vi "Supervisório Comunicação RS485.vi"() -> ()   [LabVIEW 2013]
uses:
  <vilib>/Instr/_visa.llb/VISA Configure Serial Port (Instr).vi
panel:
  in  "?":enum32{"Dados", "Gráficos"}(tab)
  out "MENSAGENS DO CONTROLADOR":string
  out "MENSAGENS DO INVERSOR":string
  out "POTENCIA SAIDA":dbl
  out "TEMPERATURA":dbl
  in  "?":bool
  in  "?":dbl(knob) scale=0.0..99.0
  in  "?":bool
  in  "?":bool
  out "STATUS DO INVERSOR":dbl
  out "POTÊNCIA DE SAÍDA [W]":dbl
  out "DC LINK [Vdc]":dbl
  out "TENSÃO DE SAÍDA [Vac]":dbl
  out "FREQUENCIA SAIDA [Hz]":dbl
  out "CORRENTE SAÍDA [A]":dbl
  in  "?":bool
  in  "Baud Rate":u32=9600
  in  "PORTA COM":refnum<visa-resource-name>
  out "?":i32(graph)
  out "?":i32(graph)
  out "?":dbl(graph)
  out "?":dbl(graph)
  out "?":dbl
  out "?":dbl
  out "?":dbl
  out "?":dbl
  # "Configura Serial"
  # "Dados do inversor"
  # "Dados temperatura"
  # "Frequencia de operação inversor"
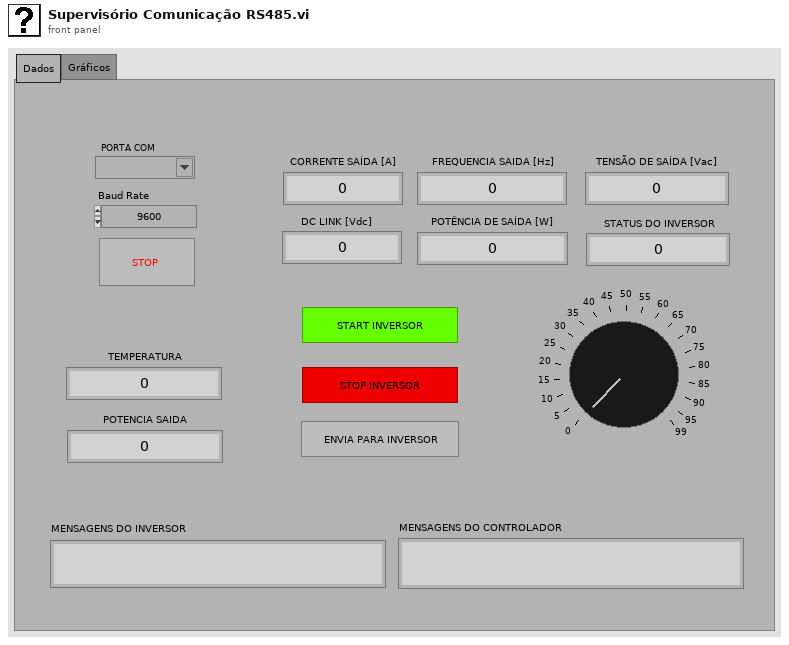
[diagram p1: front panel]
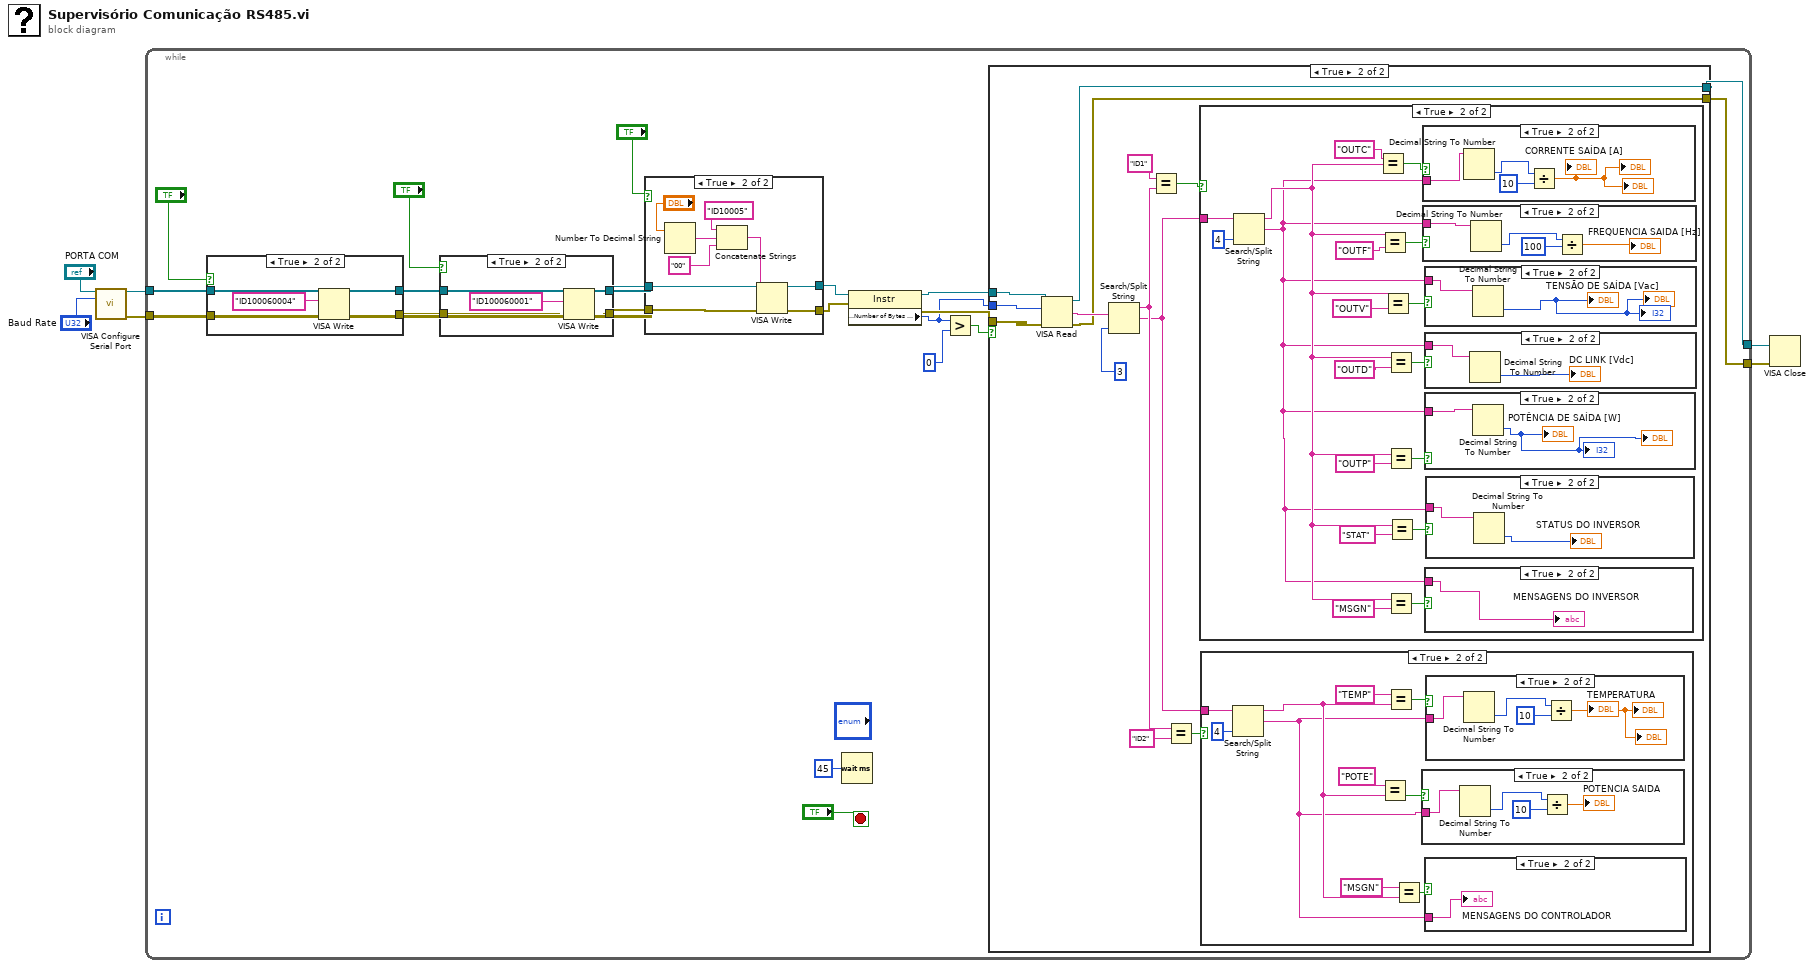
[diagram p0: block diagram]
diagram:
  n1 = call-poly "VISA Configure Serial Port"("VISA resource name"="PORTA COM", "baud rate (9600)"="Baud Rate") -> ("VISA resource name out"=w5:refnum<visa-resource-name>, "error out"=w4:errorcluster)  [unwired: 12 in]
  n2 = while {
    tunnel: w5 -> [w10]
    tunnel: w4 -> [w9]
    tunnel: [w20] -> w2
    tunnel: [w19] -> w1
    stop <- "?" stop-if-true
    n3 = case shown="True" "?" {
      tunnel: w10 -> [w28 w31]
      tunnel: w9 -> [w27 w30]
      tunnel: [w28 w32] -> w11
      tunnel: [w27 w29] -> w12
      frame False {
      }
      frame True {
        n4 = VISA Write(VISA resource name=w31, write buffer="ID100060004", error in (no error)=w30) -> (VISA resource name out=w32:refnum<visa-resource-name>, error out=w29:errorcluster)  [unwired: 1 out]
      }
    }
    n5 = case shown="True" "?" {
      tunnel: w11 -> [w46 w51]
      tunnel: w12 -> [w45 w50]
      tunnel: [w46 w48] -> w16
      tunnel: [w45 w47] -> w15
      frame False {
      }
      frame True {
        n6 = VISA Write(VISA resource name=w51, write buffer="ID100060001", error in (no error)=w50) -> (VISA resource name out=w48:refnum<visa-resource-name>, error out=w47:errorcluster)  [unwired: 1 out]
      }
    }
    n7 = case shown="True" "?" {
      tunnel: w16 -> [w35 w43]
      tunnel: w15 -> [w34 w42]
      tunnel: [w35 w37] -> w14
      tunnel: [w34 w36] -> w13
      frame False {
      }
      frame True {
        n8 = Number To Decimal String(number="?") -> (decimal integer string=w39:string)  [unwired: 1 in]
        n9 = Concatenate Strings("ID10005" ("string"), w39, "00" ("string")) -> (w41:string)
        n10 = VISA Write(VISA resource name=w43, write buffer=w41, error in (no error)=w42) -> (VISA resource name out=w37:refnum<visa-resource-name>, error out=w36:errorcluster)  [unwired: 1 out]
      }
    }
    n11 = Wait (ms)(milliseconds to wait=u32 45) -> ()  [unwired: 1 out]
    n12 = property class="Instr"(reference=w14, error in=w13) -> (reference out=w24:refnum<visa-resource-name>, error out=w23:errorcluster, "Serial Settings:Number of Bytes at Serial Port"=w22:u32)
    n13 = Greater?(x=w22, y=u32 0) -> (0:w25:bool)
    n14 = case shown="True" w25 {
      tunnel: w24 -> [w53 w55]
      tunnel: w23 -> [w52 w57]
      tunnel: w22 -> [_ w66]
      tunnel: [w53 w54] -> w20
      tunnel: [w52 w56] -> w19
      frame False {
      }
      frame True {
        n15 = VISA Read(VISA resource name=w55, byte count=w66, error in (no error)=w57) -> (VISA resource name out=w54:refnum<visa-resource-name>, read buffer=w65:string, error out=w56:errorcluster)  [unwired: 1 out]
        n16 = Search/Split String(string=w65, offset (0)=3) -> (substring before match=w60:string, match + rest of string=w58:string)  [unwired: 1 in, 1 out]
        n17 = Equal?(x="ID1", y=w60) -> (x = y?=w62:bool)
        n18 = Equal?(x=w60, y="ID2") -> (x = y?=w61:bool)
        n19 = case shown="True" w62 {
          tunnel: w58 -> [_ w103]
          frame False {
          }
          frame True {
            n20 = Search/Split String(string=w103, offset (0)=4) -> (substring before match=w87:string, match + rest of string=w86:string)  [unwired: 1 in, 1 out]
            n21 = Equal?(x="OUTC", y=w87) -> (x = y?=w100:bool)
            n22 = Equal?(x=w87, y="OUTF") -> (x = y?=w98:bool)
            n23 = Equal?(x=w87, y="OUTV") -> (x = y?=w96:bool)
            n24 = Equal?(x=w87, y="OUTD") -> (x = y?=w95:bool)
            n25 = Equal?(x=w87, y="OUTP") -> (x = y?=w93:bool)
            n26 = Equal?(x=w87, y="MSGN") -> (x = y?=w89:bool)
            n27 = Equal?(x=w87, y="STAT") -> (x = y?=w91:bool)
            n28 = case shown="True" w100 {
              tunnel: w86 -> [_ w120]
              frame False {
              }
              frame True {
                n29 = Decimal String To Number(string=w120) -> (number=w118:i32)  [unwired: 2 in, 1 out]
                n30 = Divide(x=w118, y=10) -> (x/y=→"CORRENTE SAÍDA [A]" →"?" →"?":dbl)
              }
            }
            n31 = case shown="True" w98 {
              tunnel: w86 -> [_ w116]
              frame False {
              }
              frame True {
                n32 = Decimal String To Number(string=w116) -> (number=w114:i32)  [unwired: 2 in, 1 out]
                n33 = Divide(x=w114, y=100) -> (x/y=→"FREQUENCIA SAIDA [Hz]":dbl)
              }
            }
            n34 = case shown="True" w96 {
              tunnel: w86 -> [_ w112]
              frame False {
              }
              frame True {
                n35 = Decimal String To Number(string=w112) -> (number=→"TENSÃO DE SAÍDA [Vac]" →"?" →"?":i32)  [unwired: 2 in, 1 out]
              }
            }
            n36 = case shown="True" w95 {
              tunnel: w86 -> [_ w110]
              frame False {
              }
              frame True {
                n37 = Decimal String To Number(string=w110) -> (number=→"DC LINK [Vdc]":i32)  [unwired: 2 in, 1 out]
              }
            }
            n38 = case shown="True" w93 {
              tunnel: w86 -> [_ w108]
              frame False {
              }
              frame True {
                n39 = Decimal String To Number(string=w108) -> (number=→"POTÊNCIA DE SAÍDA [W]" →"?" →"?":i32)  [unwired: 2 in, 1 out]
              }
            }
            n40 = case shown="True" w89 {
              tunnel: w86 -> [_ w104]
              frame False {
              }
              frame True {
                "MENSAGENS DO INVERSOR" <- w104
              }
            }
            n41 = case shown="True" w91 {
              tunnel: w86 -> [_ w106]
              frame False {
              }
              frame True {
                n42 = Decimal String To Number(string=w106) -> (number=→"STATUS DO INVERSOR":i32)  [unwired: 2 in, 1 out]
              }
            }
          }
        }
        n43 = case shown="True" w61 {
          tunnel: w58 -> [_ w76]
          frame False {
          }
          frame True {
            n44 = Search/Split String(string=w76, offset (0)=4) -> (substring before match=w69:string, match + rest of string=w67:string)  [unwired: 1 in, 1 out]
            n45 = Equal?(x="POTE", y=w69) -> (x = y?=w70:bool)
            n46 = Equal?(x="TEMP", y=w69) -> (x = y?=w73:bool)
            n47 = Equal?(x="MSGN", y=w69) -> (x = y?=w72:bool)
            n48 = case shown="True" w70 {
              tunnel: w67 -> [_ w80]
              frame False {
              }
              frame True {
                n49 = Decimal String To Number(string=w80) -> (number=w78:i32)  [unwired: 2 in, 1 out]
                n50 = Divide(x=w78, y=10) -> (x/y=→"POTENCIA SAIDA":dbl)
              }
            }
            n51 = case shown="True" w72 {
              tunnel: w67 -> [_ w81]
              frame False {
              }
              frame True {
                "MENSAGENS DO CONTROLADOR" <- w81
              }
            }
            n52 = case shown="True" w73 {
              tunnel: w67 -> [_ w85]
              frame False {
              }
              frame True {
                n53 = Decimal String To Number(string=w85) -> (number=w83:i32)  [unwired: 2 in, 1 out]
                n54 = Divide(x=w83, y=10) -> (x/y=→"TEMPERATURA" →"?" →"?":dbl)
              }
            }
          }
        }
      }
    }
  }
  n55 = VISA Close(VISA resource name=w2, error in (no error)=w1) -> ()  [unwired: 1 out]
